vi "Verify Configuration.vi"(0 "eye scan in":refnum<class "niHighSpeedSerial Eye Scan v1 Host.lvclass">, 11 "error in":errorcluster) -> (4 "eye scan out":refnum<class "niHighSpeedSerial Eye Scan v1 Host.lvclass">, 15 "error out":errorcluster)   [LabVIEW 2014, in "niHighSpeedSerial Eye Scan v1 Host.lvclass"]
doc: "Validates that the current configuration is valid before starting Eye Scan on the FPGA.\n\n<B>Input Parameters</B>\n\n<B>eye scan in</B> Takes in a reference to your session from the previous VI.\n\n<B>error in</B> describes error conditions that occur before this node runs. This input provides standard 'error in' functionality.\n\n<B>Output Parameters</B>\n\n<B>eye scan out</B> passes a reference to your session to the next VI.\n\n<B>error out</B> contains error information. This output provides standard 'error out' functionality."
uses:
  <instrlib>/niHighSpeedSerial/Eye Scan/v1/Host/Eye Scan/niHighSpeedSerial Eye Scan v1 Host.lvclass
  <instrlib>/niHighSpeedSerial/Eye Scan/v1/Host/Eye Scan/niHighSpeedSerial Eye Scan v1 Host.lvclass/niHighSpeedSerial Eye Scan v1 Host.ctl
  <vilib>/Utility/error.llb/Error Cluster From Error Code.vi
  <vilib>/ErrorRing/Error Ring.xnode
  <instrlib>/niHighSpeedSerial/Eye Scan/v1/Host/Common/niHighSpeedSerial Eye Scan Common v1 Host.lvlib
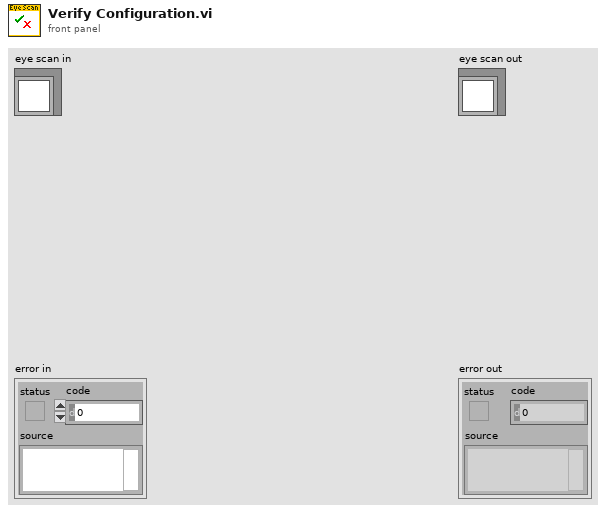
[diagram p1: front panel]
types:
  T1 = typedef "niHighSpeedSerial Eye Scan v1 Host.lvclass/Private Data.ctl" = cluster{"instruction target":refnum<class "niInstr Instruction Target v1 Host.lvclass">, "channels":T2[], "measure state":T3, "rx output divider":T4, "equalization mode":T5, "rx data width":T6, "BER floor":dbl, "number of points completed":i32, "rx output divider configured?":bool, "equalization mode configured?":bool, "rx data width configured?":bool}
  T2 = typedef "niHighSpeedSerial Eye Scan v1 Host.lvclass/Channel Data.ctl" = cluster{"instance":u8, "channel":refnum<class "niHighSpeedSerial Eye Scan Single Point v1 Host.lvclass">, "point iterator":refnum<class "niHighSpeedSerial Eye Scan Point Iterator v1 Host.lvclass">}
  T3 = typedef "niHighSpeedSerial Eye Scan v1 Host.lvclass/Measure State.ctl" = enum16{"Uninitialized", "Initialized", "Ready", "Measuring", "Finished", "Aborted"}
  T4 = typedef "niHighSpeedSerial Eye Scan Common v1 Host.lvlib/RX Output Divider.ctl" = enum16{"1", "2", "4", "8", "16"}
  T5 = typedef "niHighSpeedSerial Eye Scan Common v1 Host.lvlib/Equalization Mode.ctl" = enum16{"DFE", "LPM"}
  T6 = typedef "niHighSpeedSerial Eye Scan Common v1 Host.lvlib/Data Width.ctl" = enum16{"16 Bit", "20 Bit", "32 Bit", "40 Bit"}
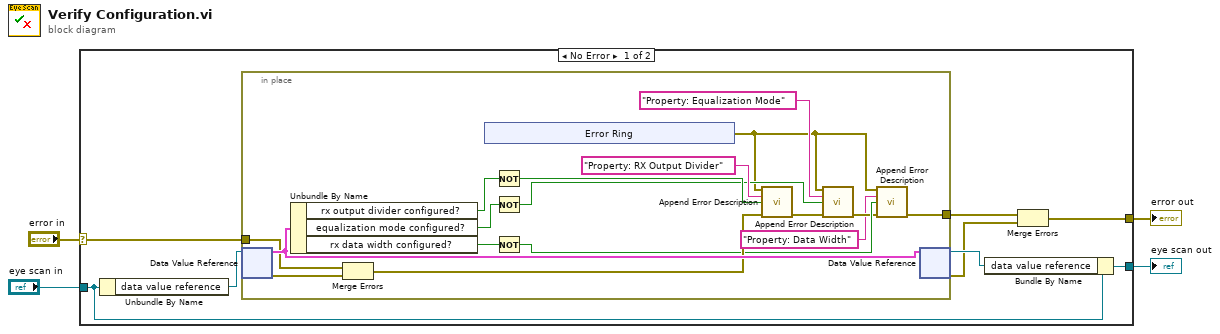
[diagram p0: block diagram]
diagram:
  n1 = case shown="No Error" "error in" {
    selector: "error in" -> [w7 w35]
    tunnel: [w6 w35] -> w3
    tunnel: [w12 w34] -> w1
    tunnel: "eye scan in" -> [w11 w34]
    frame No Error {
      n2 = Unbundle By Name(w11) -> ("data value reference"=w10:refnum<data-value>)
      n3 = in-place {
        in-place-border: w7 -> [w28]
        in-place-border: [w14] -> w5
        n4 = in-place-dvr #1(w10) -> (w29:T1, w27:errorcluster)
        n5 = Unbundle By Name(w29) -> ("rx output divider configured?"=w24:bool, "equalization mode configured?"=w20:bool, "rx data width configured?"=w17:bool)
        n6 = Merge Errors(w28, w27) -> (w26:errorcluster)
        n7 = xnode "Error Ring"() -> ("error out"=w18:errorcluster)
        n8 = Not(x=w24) -> (.not. x?=w23:bool)
        n9 = Not(x=w20) -> (.not. x?=w19:bool)
        n10 = Not(x=w17) -> (.not. x?=w16:bool)
        n11 = call <instrlib>:"Append Error Description.vi"("error to append"=w18, "append string (\"\")"="Property: RX Output Divider" ("append string (\"\")"), "generate error?"=w23, "error in"=w26) -> ("error out"=w21:errorcluster)  [unwired: 11 in]
        n12 = call <instrlib>:"Append Error Description.vi"("error to append"=w18, "append string (\"\")"="Property: Equalization Mode" ("append string (\"\")"), "generate error?"=w19, "error in"=w21) -> ("error out"=w15:errorcluster)  [unwired: 11 in]
        n13 = call <instrlib>:"Append Error Description.vi"("error to append"=w18, "append string (\"\")"="Property: Data Width" ("append string (\"\")"), "generate error?"=w16, "error in"=w15) -> ("error out"=w14:errorcluster)  [unwired: 11 in]
        n14 = in-place-dvr #1(w29) -> (w9:refnum<data-value>, w8:errorcluster)
      }
      n15 = Bundle By Name(cluster=w11, "data value reference"=w9) -> (w12:refnum<class "niHighSpeedSerial Eye Scan v1 Host.lvclass">)
      n16 = Merge Errors(w5, w8) -> (w6:errorcluster)
    }
    frame Error {
    }
  }
  "error out" <- w3
  "eye scan out" <- w1
